vi "HIOKI PW3390 Conf CH B Pulse.vi"(0 "VISA Resource":refnum<visa-resource-name>, 1 "Unit (2: rpm)":enum16{"V", "Hz", "rpm"}(ring)=enum."rpm", 2 "Max Frequency (3: 5kHz)":enum16{"100Hz", "500Hz", "1kHz", "5kHz"}(ring)=enum."5kHz", 3 "Number (2)":i32=2 min=1 max=60000, 4 "Motorpoles (4)":i32=4 min=2 max=98 step=2, 5 "error in (no error)":errorcluster, 6 "Set/Query (F: Set)":bool, 7 "CH Z input (0: OFF)":enum16{"OFF", "ON", "BPHASE"}(ring), 9 "OPC query (T: ON)":bool=TRUE, 11 "Error Out (F: Off)":bool) -> (12 "CH B input out":enum16{"PULSE", "DC"}(ring), 13 "CH Z input out":enum16{"OFF", "ON", "BPHASE"}(ring), 14 "VISA Resource out":refnum<visa-resource-name>, 15 "Unit out":enum16{"V", "Hz", "rpm"}(ring)=enum."rpm", 16 "Max Frequency out":enum16{"100Hz", "500Hz", "1kHz", "5kHz"}(ring)=enum."5kHz", 17 "Number out":i32=2, 18 "Motorpoles out":i32=4, 19 "error out":errorcluster)   [LabVIEW 2009]
doc: "Sets and reads the functions related to the Motor Analysis Option's Channel B pulse.\n\nSet/Query\n Set: Send the setting commands for the device.\n Query: Query the setting of the device.\n\nUnit\n Sets the unit of Channel B.\n \nMax Frequency\n Sets the measured maximum frequency of Channel B.\n\nNumber\n Sets the pulse value of Channel B. Only half multiples of the motor poles that are set can be set.\n Input Range: 1 - 60000\n\nMotorpoles\n Sets the motor poles. When an odd number is set, an even number smaller than the set value will be set.\n Input Range: even values of 2 - 98\n\nCH Z input\n Sets the Channel Z Input."
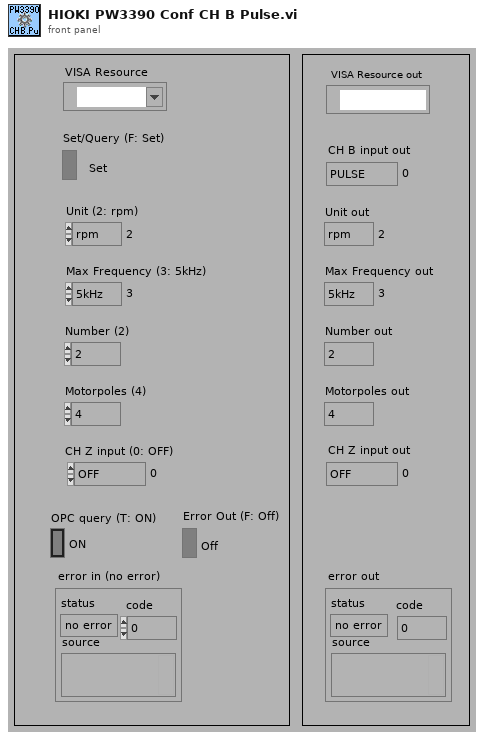
[diagram p1: front panel]
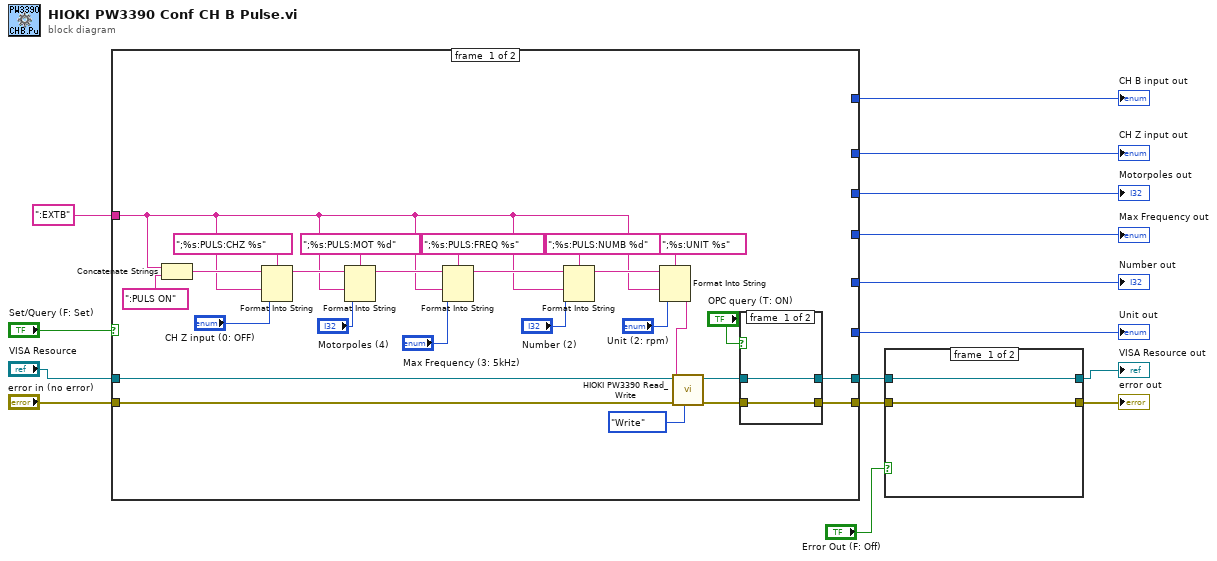
[diagram p0: block diagram]
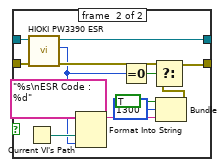
[diagram p2: hidden frame]
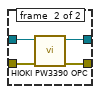
[diagram p3: hidden frame]
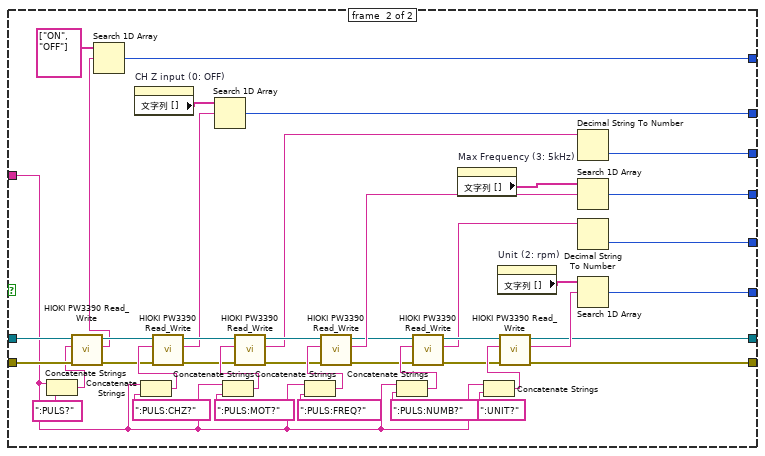
[diagram p4: hidden frame]
diagram:
  n1 = case shown="FALSE" "Set/Query (F: Set)" {
    tunnel: "error in (no error)" -> [w38 w56]
    tunnel: [w19 w74] -> w6
    tunnel: "VISA Resource" -> [w39 w57]
    tunnel: [w20 w75] -> w5
    tunnel: [_ w73] -> w13
    tunnel: ":EXTB" -> [w17 w53]
    tunnel: [_ w65] -> w11
    tunnel: [_ w87] -> w10
    tunnel: [_ w61] -> w8
    tunnel: [_ w60] -> w9
    tunnel: [_ w48] -> w1
    frame #0 {
      n2 = Concatenate Strings(w17, ":PULS ON") -> (w18:string)
      n3 = Format Into String(format string=";%s:PULS:CHZ %s", initial string=w18, w17, "CH Z input (0: OFF)") -> (resulting string=w25:string)  [unwired: 1 in, 1 out]
      n4 = Format Into String(format string=";%s:PULS:MOT %d", initial string=w25, w17, "Motorpoles (4)") -> (resulting string=w35:string)  [unwired: 1 in, 1 out]
      n5 = Format Into String(format string=";%s:PULS:FREQ %s", initial string=w35, w17, "Max Frequency (3: 5kHz)") -> (resulting string=w26:string)  [unwired: 1 in, 1 out]
      n6 = Format Into String(format string=";%s:PULS:NUMB %d", initial string=w26, w17, "Number (2)") -> (resulting string=w29:string)  [unwired: 1 in, 1 out]
      n7 = Format Into String(format string=";%s:UNIT %s", initial string=w29, w17, "Unit (2: rpm)") -> (resulting string=w24:string)  [unwired: 1 in, 1 out]
      n8 = call <instrlib>:"HIOKI PW3390 Read_Write.vi"("Read/Write"=enum16{"Read", "Write"}."Write", "error in (no error)"=w38, "data in"=w24, "VISA Resource"=w39) -> ("error out"=w21:errorcluster, "VISA Resource out"=w22:refnum<visa-resource-name>)  [unwired: 5 in, 1 out]
      n9 = case shown="TRUE" "OPC query (T: ON)" {
        tunnel: [w43 w47] -> w20
        tunnel: [w42 w46] -> w19
        tunnel: w22 -> [w43 w45]
        tunnel: w21 -> [w42 w44]
        frame #0 {
        }
        frame #1 {
          n10 = call <instrlib>:"HIOKI PW3390 OPC.vi"("error in (no error)"=w44, "VISA Resource"=w45) -> ("error out"=w46:errorcluster, "VISA Resource out"=w47:refnum<visa-resource-name>)  [unwired: 7 in, 1 out]
        }
      }
    }
    frame #1 {
      n11 = Concatenate Strings(w53, ":PULS?" ("文字列")) -> (w51:string)
      n12 = call <instrlib>:"HIOKI PW3390 Read_Write.vi"("error in (no error)"=w56, "data in"=w51, "VISA Resource"=w57) -> ("error out"=w54:errorcluster, "data out"=w49:string, "VISA Resource out"=w55:refnum<visa-resource-name>)  [unwired: 6 in]
      n13 = Search 1D Array(1D array=string[] ["ON", "OFF"] ("文字列配列"), element=w49) -> (index of element=w48:i32)  [unwired: 1 in]
      n14 = property on="CH Z input (0: OFF)" class="Enum （指定）"() -> ("文字列 []"=w58:string[])  [unwired: 2 in, 2 out]
      n15 = Concatenate Strings(w53, ":PULS:CHZ?") -> (w71:string)
      n16 = call <instrlib>:"HIOKI PW3390 Read_Write.vi"("error in (no error)"=w54, "data in"=w71, "VISA Resource"=w55) -> ("error out"=w68:errorcluster, "data out"=w59:string, "VISA Resource out"=w69:refnum<visa-resource-name>)  [unwired: 6 in]
      n17 = Search 1D Array(1D array=w58, element=w59) -> (index of element=w60:i32)  [unwired: 1 in]
      n18 = Concatenate Strings(w53, ":PULS:MOT?") -> (w82:string)
      n19 = call <instrlib>:"HIOKI PW3390 Read_Write.vi"("error in (no error)"=w68, "data in"=w82, "VISA Resource"=w69) -> ("error out"=w84:errorcluster, "data out"=w72:string, "VISA Resource out"=w85:refnum<visa-resource-name>)  [unwired: 6 in]
      n20 = Concatenate Strings(w53, ":PULS:FREQ?") -> (w86:string)
      n21 = call <instrlib>:"HIOKI PW3390 Read_Write.vi"("error in (no error)"=w84, "data in"=w86, "VISA Resource"=w85) -> ("error out"=w63:errorcluster, "data out"=w66:string, "VISA Resource out"=w64:refnum<visa-resource-name>)  [unwired: 6 in]
      n22 = Concatenate Strings(w53, ":PULS:NUMB?") -> (w78:string)
      n23 = call <instrlib>:"HIOKI PW3390 Read_Write.vi"("error in (no error)"=w63, "data in"=w78, "VISA Resource"=w64) -> ("error out"=w76:errorcluster, "data out"=w62:string, "VISA Resource out"=w77:refnum<visa-resource-name>)  [unwired: 6 in]
      n24 = property on="Max Frequency (3: 5kHz)" class="Enum (strict)"() -> ("文字列 []"=w67:string[])  [unwired: 2 in, 2 out]
      n25 = Concatenate Strings(w53, ":UNIT?") -> (w83:string)
      n26 = property on="Unit (2: rpm)" class="Enum (strict)"() -> ("文字列 []"=w81:string[])  [unwired: 2 in, 2 out]
      n27 = call <instrlib>:"HIOKI PW3390 Read_Write.vi"("error in (no error)"=w76, "data in"=w83, "VISA Resource"=w77) -> ("error out"=w74:errorcluster, "data out"=w80:string, "VISA Resource out"=w75:refnum<visa-resource-name>)  [unwired: 6 in]
      n28 = Decimal String To Number(string=w72) -> (number=w73:i32)  [unwired: 2 in, 1 out]
      n29 = Search 1D Array(1D array=w67, element=w66) -> (index of element=w65:i32)  [unwired: 1 in]
      n30 = Decimal String To Number(string=w62) -> (number=w61:i32)  [unwired: 2 in, 1 out]
      n31 = Search 1D Array(1D array=w81, element=w80) -> (index of element=w87:i32)  [unwired: 1 in]
    }
  }
  "Motorpoles out" <- w13
  "Unit out" <- w10
  "Max Frequency out" <- w11
  "Number out" <- w8
  "CH Z input out" <- w9
  "CH B input out" <- w1
  n32 = case shown="TRUE" "Error Out (F: Off)" {
    tunnel: w5 -> [w92 w105]
    tunnel: w6 -> [w91 w104]
    tunnel: [w91 w94] -> w4
    tunnel: [w92 w103] -> w2
    frame #0 {
    }
    frame #1 {
      n33 = Current VI's Path() -> (path=w101:path)
      n34 = call <instrlib>:"HIOKI PW3390 ESR.vi"("error in (no error)"=w104, "VISA Resource"=w105) -> ("error out"=w95:errorcluster, "Output Value"=w93:u8, "VISA Resource out"=w103:refnum<visa-resource-name>)  [unwired: 6 in, 1 out]
      n35 = Format Into String(format string="%s\nESR Code : %d", w101, w93) -> (resulting string=w97:string)  [unwired: 2 in, 1 out]
      n36 = Equal To 0?(x=w93) -> (x = 0?=w102:bool)
      n37 = Bundle("status"=TRUE, "code"=1300, w97) -> (w96:cluster{"status":bool, "code":i32, string})  [unwired: 1 in]
      n38 = Select(t=w95, s=w102, f=w96) -> (s? t:f=w94:errorcluster)
    }
  }
  "error out" <- w4
  "VISA Resource out" <- w2
